vi "Exemple de mesure.vi"() -> ()   [LabVIEW 2013]
panel:
  out "XY Graph":cluster{dbl[], dbl[]}(graph)
  out "P1/P2":dbl format="%#_13g"
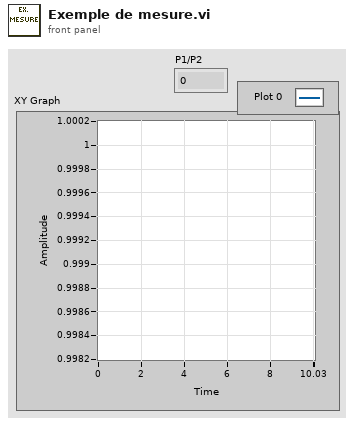
[diagram p1: front panel]
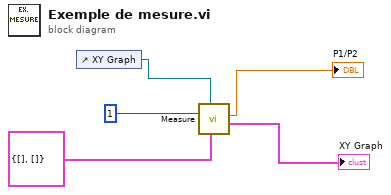
[diagram p0: block diagram]
diagram:
  n1 = control-ref of="XY Graph"() -> (w2:refnum<vi>)
  n2 = call "Measure.vi"("Graph in"=cluster{dbl[], dbl[]} {[], []}, "XY Graph"=w2, "Reference Cell"=1) -> ("Values"=→"XY Graph":cluster{dbl[], dbl[]}, "P1/P2"=→"P1/P2":dbl)  [unwired: 6 in, 1 out]
